vi "欧姆龙PLC通讯Fans UDP-读PLC寄存器编码.vi"(9 "读取寄存器个数":u16, 11 "起始地址16":string) -> (3 "读PLC寄存器编码字符串":string)   [LabVIEW 2014]
panel:
  out "16bit寄存器个数":string
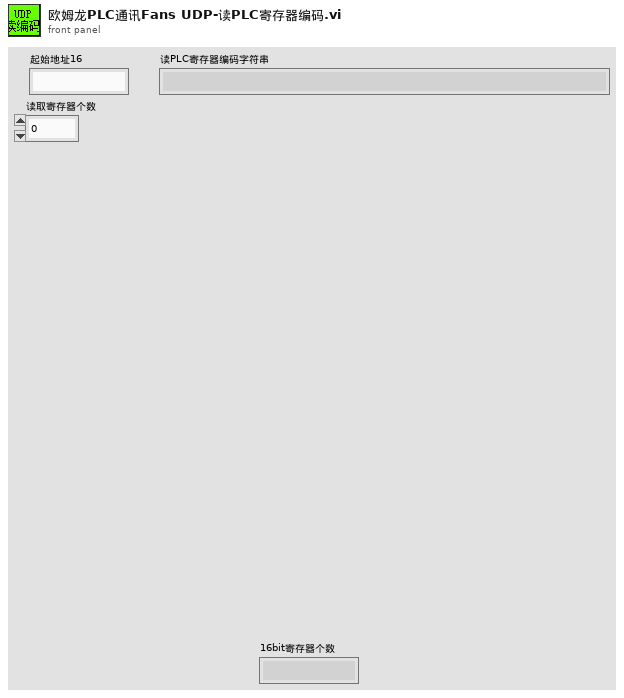
[diagram p1: front panel]
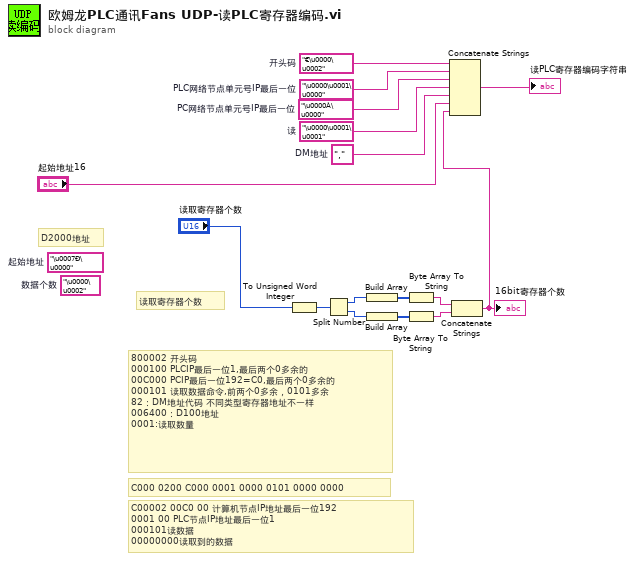
[diagram p0: block diagram]
diagram:
  (unwired) "\u0007Ð\u0000"  # 起始地址
  (unwired) "\u0000\u0002"  # 数据个数
  w14 = "‚"  # DM地址
  w13 = "\u0000\u0001\u0001"  # 读
  w12 = "\u0000À\u0000"  # PC网络节点单元号IP最后一位
  w11 = "\u0000\u0001\u0000"  # PLC网络节点单元号IP最后一位
  w10 = "€\u0000\u0002"  # 开头码
  # "读取寄存器个数"
  # "C000 0200 C000 0001 0000 0101 0000 0000"
  # "C00002 00C0 00 计算机节点IP地址最后一位192\n0001 00 PLC节点IP地址最后一位1\n000101读数据\n00000000读取到的数据"
  # "800002 开头码\n000100 PLCIP最后一位1,最后两个0多余的\n00C000 PCIP最后一位192=C0,最后两个0多余的\n000101 读取数据命令,前两个0多余，0101多余\n82：DM地址代码 不同类型寄存器地址不一样\n006400：D100地址\n0001:读取数量"
  # "D2000地址"
  n1 = To Unsigned Word Integer(number="读取寄存器个数") -> (unsigned 16bit integer=w3:u16)
  n2 = Split Number(x=w3) -> (hi(x)=w4:u8, lo(x)=w5:u8)
  n3 = Build Array(w4) -> (w6:u8[])
  n4 = Build Array(w5) -> (w7:u8[])
  n5 = Byte Array To String(unsigned byte array=w6) -> (string=w8:string)
  n6 = Byte Array To String(unsigned byte array=w7) -> (string=w9:string)
  n7 = Concatenate Strings(w8, w9) -> (w1:string)
  "16bit寄存器个数" <- w1
  n8 = Concatenate Strings(w10, w11, w12, w13, w14, "起始地址16", w1) -> (→"读PLC寄存器编码字符串":string)
